vi "T7_Write_UINT16_Register.vi"(0 "Remote IP Address":string="192.168.124.53", 1 "Remote Port":u16=502, 2 "FirstChannel":u16, 3 "error in (no error)":errorcluster, 4 "UINT16 to Write":u16=1) -> (9 "WrittenAt":timestamp=timestamp(3519914743.248914 s since 1904-01-01), 10 "error out":errorcluster)   [LabVIEW 2015]
uses:
  Serial Link Layer/NI_Modbus_Cleaned/NI Modbus121Clean.llb/MB Ethernet Master Query Write Multiple Registers (poly).vi
panel:
  out "Starting Address":u16=2000
  # "MB Ethernet Example Master.vi\n\nInstructions\n1.Use Kipling to find your devices IP address & modify the\n\"Remote IP Addres\"\n2. Run this VI\n3. Change value of \"UINT16 to Write\" & press \"Write Data\""
  # "TCP Parameters"
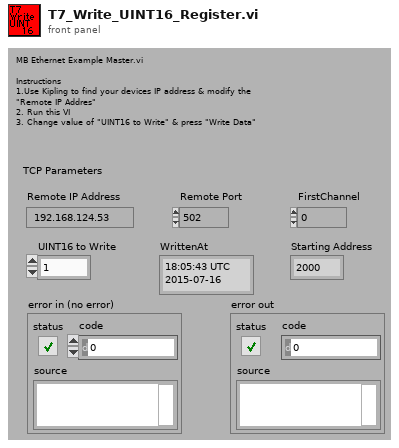
[diagram p1: front panel]
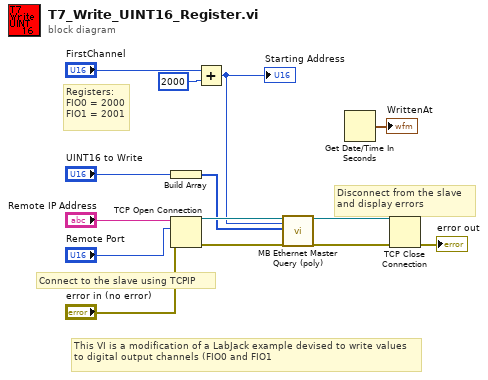
[diagram p0: block diagram]
diagram:
  # "This VI is a modification of a LabJack example devised to write values to digital output channels (FIO0 and FIO1"
  # "Registers:\nFIO0 = 2000\nFIO1 = 2001"
  # "Disconnect from the slave\nand display errors"
  # "Connect to the slave using TCPIP"
  n1 = Build Array("UINT16 to Write") -> (w8:u16[])
  n2 = TCP Open Connection(address="Remote IP Address", remote port or service name="Remote Port", error in (no error)="error in (no error)") -> (connection ID=w12:refnum<k5>, error out=w11:errorcluster)  [unwired: 2 in]
  n3 = Add(x="FirstChannel", y=2000) -> (x+y=w5:i32)
  "Starting Address" <- w5
  n4 = call-poly "MB Ethernet Master Query (poly).vi"("TCP Connection Refnum in"=w12, "Starting Address"=w5, "Registers"=w8, "error in"=w11) -> ("TCP Connection Refnum (dup)"=w10:refnum<k5>, "error out"=w9:errorcluster)  [unwired: 13 in, 1 out]
  n5 = Get Date/Time In Seconds() -> (seconds since 1Jan1904=→"WrittenAt":timestamp)
  n6 = TCP Close Connection(connection ID=w10, error in (no error)=w9) -> (error out=→"error out":errorcluster)  [unwired: 2 out]
